vi "Servo-Motor_Tset.vi"() -> ()   [LabVIEW 2019]
panel:
  in  "角度 2":dbl
  in  "Stop":bool
  in  "角度":dbl(knob) scale=0.0..180.0
  in  "伺服馬達角位 2":tag="B/PWM2"
  in  "伺服馬達角位":tag="A/PWM2"
  in  "Error In":errorcluster
  out "error out":errorcluster
  # "180"
  # "50"
  # "110.5"
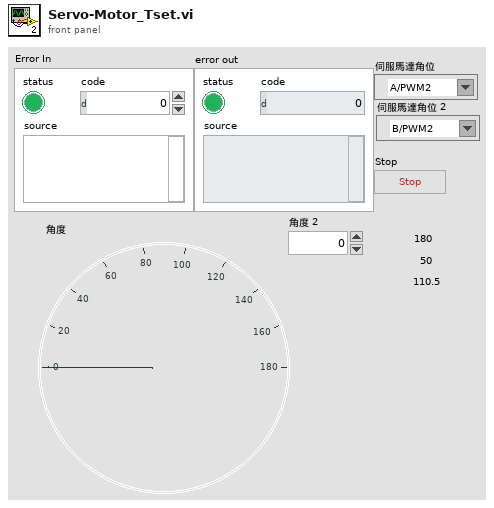
[diagram p1: front panel]
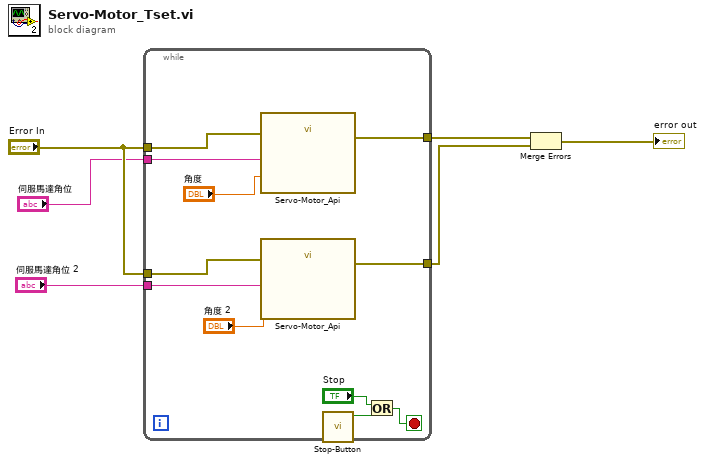
[diagram p0: block diagram]
diagram:
  n1 = while {
    tunnel: [w17] -> w6
    tunnel: [w16] -> w5
    tunnel: "Error In" -> [w15]
    tunnel: "Error In" -> [w14]
    tunnel: "伺服馬達角位" -> [w13]
    tunnel: "伺服馬達角位 2" -> [w12]
    stop <- w9 stop-if-true
    n2 = call "Servo-Motor_Api.vi"("角度"="角度", "Error In"=w15, "伺服馬達角位"=w13) -> ("Error Out"=w17:errorcluster)  [unwired: 8 in]
    n3 = call "Servo-Motor_Api.vi"("角度"="角度 2", "Error In"=w14, "伺服馬達角位"=w12) -> ("Error Out"=w16:errorcluster)  [unwired: 8 in]
    n4 = call "Stop-Button.vi"() -> ("顯示按下?"=w11:bool)  [unwired: 10 in, 1 out]
    n5 = Or(x="Stop", y=w11) -> (x .or. y?=w9:bool)
  }
  n6 = Merge Errors(w6, w5) -> (→"error out":errorcluster)
